vi "read txt.vi"() -> (2 "selected path":path caption="선택된 경로", 3 "Output":string)   [LabVIEW 2015]
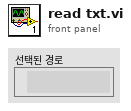
[diagram p1: front panel]
types:
  T1 = enum16{"open", "replace", "create", "open or create", "replace or create", "replace or create with confirmation"}
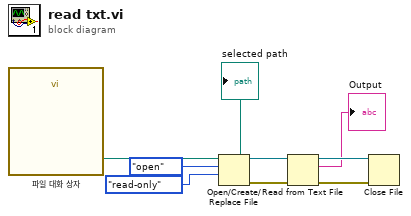
[diagram p0: block diagram]
diagram:
  n1 = call "파일 대화 상자"() -> ("selected path"=w8:path)  [unwired: 12 in, 3 out]
  "selected path" <- w8
  n2 = Open/Create/Replace File(file path (use dialog)=w8, operation (0:open)=T1."open" ("동작(0:open)"), access (0:read/write)=enum16{"read/write", "read-only", "write-only"}."read-only" ("접근(0:읽기/쓰기)")) -> (refnum out=w7:refnum<file>, error out=w5:errorcluster)  [unwired: 3 in, 1 out]
  n3 = Read from Text File(file (use dialog)=w7, error in=w5) -> (refnum out=w6:refnum<file>, text=→"Output":string, error out=w4:errorcluster)  [unwired: 2 in, 1 out]
  n4 = Close File(refnum=w6, error in=w4) -> ()  [unwired: 2 out]
